vi "RSZVB Set Time Gate State.vi"(8 "error in (no error)":errorcluster {"code" format="%.0x"}, 9 "Time Gate (F: Off)":bool, 10 "Channel (Trace) (1)":i32=1, 11 "VISA session":refnum<visa-resource-name>) -> (0 "error out":errorcluster {"code" format="%.0x"}, 3 "dup VISA session":refnum<visa-resource-name>)   [LabVIEW 2011]
doc: "This VI determines whether the time gate for trace no. <Ch/Tr> is enabled.\n\nRemote-control command(s):\nCALCulate<Ch/Tr>:FILTer[:GATE]:TIME:STATe ON | OFF"
panel:
  # "On\nOff"
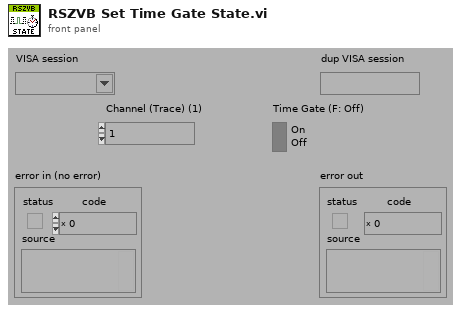
[diagram p1: front panel]
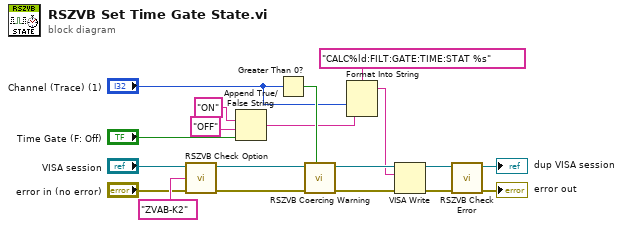
[diagram p0: block diagram]
diagram:
  n1 = call "RSZVB Check Option.vi"("error in (no error)"="error in (no error)", "Options"="ZVAB-K2", "VISA session"="VISA session") -> ("error out"=w8:errorcluster, "dup VISA session"=w7:refnum<visa-resource-name>)  [unwired: 7 in]
  n2 = Append True/False String(1:"Time Gate (F: Off)", 2:"OFF", 3:"ON") -> (0:w10:string)  [unwired: 1 in]
  n3 = Greater Than 0?(x="Channel (Trace) (1)") -> (x > 0?=w11:bool)
  n4 = call "RSZVB Coercing Warning.vi"("In Range?"=w11, "error in (no error)"=w8, "VISA session"=w7) -> ("error out"=w15:errorcluster, "dup VISA session"=w16:refnum<visa-resource-name>)  [unwired: 7 in]
  n5 = Format Into String(format string="CALC%ld:FILT:GATE:TIME:STAT %s", "Channel (Trace) (1)", w10) -> (resulting string=w12:string)  [unwired: 2 in, 1 out]
  n6 = VISA Write(VISA resource name=w16, write buffer=w12, error in (no error)=w15) -> (VISA resource name out=w13:refnum<visa-resource-name>, error out=w14:errorcluster)  [unwired: 1 out]
  n7 = call "RSZVB Check Error.vi"("error in (no error)"=w14, "VISA session"=w13) -> ("error out"=→"error out":errorcluster, "dup VISA session"=→"dup VISA session":refnum<visa-resource-name>)  [unwired: 8 in]
